vi "Set Cursor.vi"(8 "error in (no error)":errorcluster, 10 "position":cluster{"row":i8, "column":i8}, 11 "LCD in":refnum<class "Character LCD.lvclass">) -> (0 "error out":errorcluster, 3 "LCD out":refnum<class "Character LCD.lvclass">)   [LabVIEW 2015, in "HD44780 Host.lvlib"]
uses:
  HD44780 Host.lvlib
  Internal/LCD Class/Character LCD.lvclass
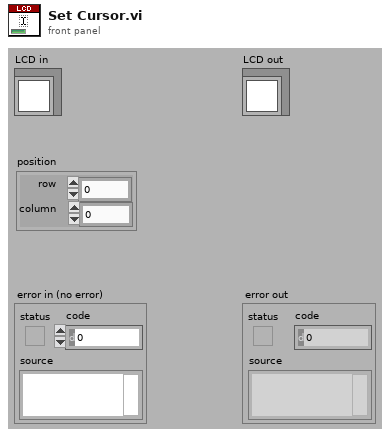
[diagram p1: front panel]
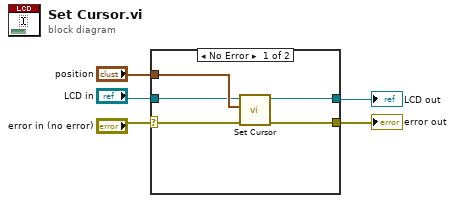
[diagram p0: block diagram]
diagram:
  n1 = case shown="No Error" "error in (no error)" {
    selector: "error in (no error)" -> [w9 w12]
    tunnel: [w7 w12] -> w3
    tunnel: "position" -> [w10 _]
    tunnel: "LCD in" -> [w8 w11]
    tunnel: [w6 w11] -> w1
    frame No Error {
      n2 = call-dynamic "Set Cursor.vi"("error in (no error)"=w9, "position"=w10, "Character LCD in"=w8) -> ("error out"=w7:errorcluster, "Character LCD out"=w6:refnum<class "Character LCD.lvclass">)  [unwired: 7 in]
    }
    frame Error {
    }
  }
  "error out" <- w3
  "LCD out" <- w1
